vi "WaitForEdge_SingleChannel.vi"(4 "Timeout (msec)":i32, 5 "Edge":enum16{"Rising", "Falling", "Both"}(ring), 6 "Bounce time (msec)":i32, 7 "Channel":i32, 8 "error in":errorcluster) -> (0 "error out":errorcluster, 3 "Channel out":i32)   [LabVIEW 2014]
doc: "Waits for a specified edge the input channel. Channel out is the input channel if an edge is detected, or -1 if the wait times out.\n\nThe channel must be configured as an input before calling this VI."
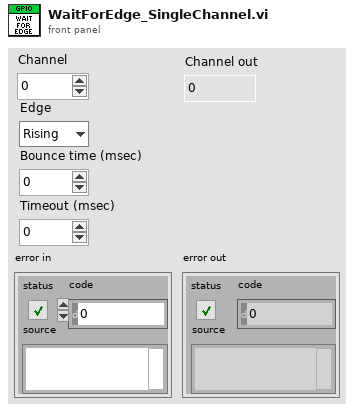
[diagram p1: front panel]
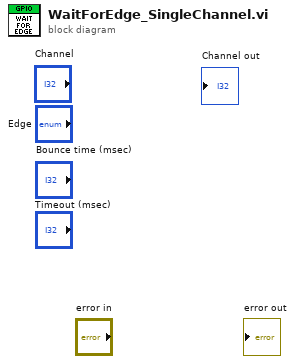
[diagram p0: block diagram]
diagram:
